vi "main_real-time control mouse 23.3.1.vi"() -> ()   [LabVIEW 2020]
uses:
  <vilib>/Analysis/3filter.llb/Filter Passband Type.ctl
  <vilib>/Analysis/NI_AALBase.lvlib
  <vilib>/Analysis/3filter.llb/Butterworth Filter (DBL).vi
  <vilib>/express/express analysis/Spectral/XNode/ExpressSpectralMeasurementsBlockNode.xnode
  <vilib>/express/express analysis/Spectral/Block/exnSpectralBlock spectral measurements power poly.vi
  <vilib>/Analysis/NI_AALPro.lvlib
  <vilib>/Analysis/NI_AAL_SigProc.lvlib
  <vilib>/Utility/file.llb/Write Delimited Spreadsheet (DBL).vi
  <vilib>/express/express analysis/Spectral/Block/exnSpectralBlock spectral measurements power DDT.vi
panel:
  out "手势":string
  in  "训练——手势":string
  out "卡尔曼滤波":cluster{"Y":dbl[], "Y":dbl[]}[](graph)
  out "通道1":dynamicdata(graph)
  out "XY Graph 2":cluster{"Y":dbl[], "Y":dbl[]}[](graph) caption="ML_集成树"
  in  "训练——位置":dbl
  out "数值":dbl
  out "采样点 2":dbl
  out "采样点":dbl
  out "ToF 2(cm)":dbl
  out "ToF 1(cm)":dbl
  out "有手势":bool
  out "最大值 1":dbl
  out "最大值2":dbl
  out "波形图 2":dbl[](graph)
  out "余数 2":dbl
  out "循环 2":dbl
  out "波形图":dbl[](graph)
  out "通道1_去环境噪声":dbl[](graph)
  out "通道2_去环境+滤波":dbl[](graph)
  out "频谱2":dynamicdata(graph)
  out "通道1_滤波":dbl[](graph)
  out "通道2_滤波":dbl[](graph)
  out "激励信号":dynamicdata(graph)
  out "通道2":dynamicdata(graph)
  in  "停止":bool
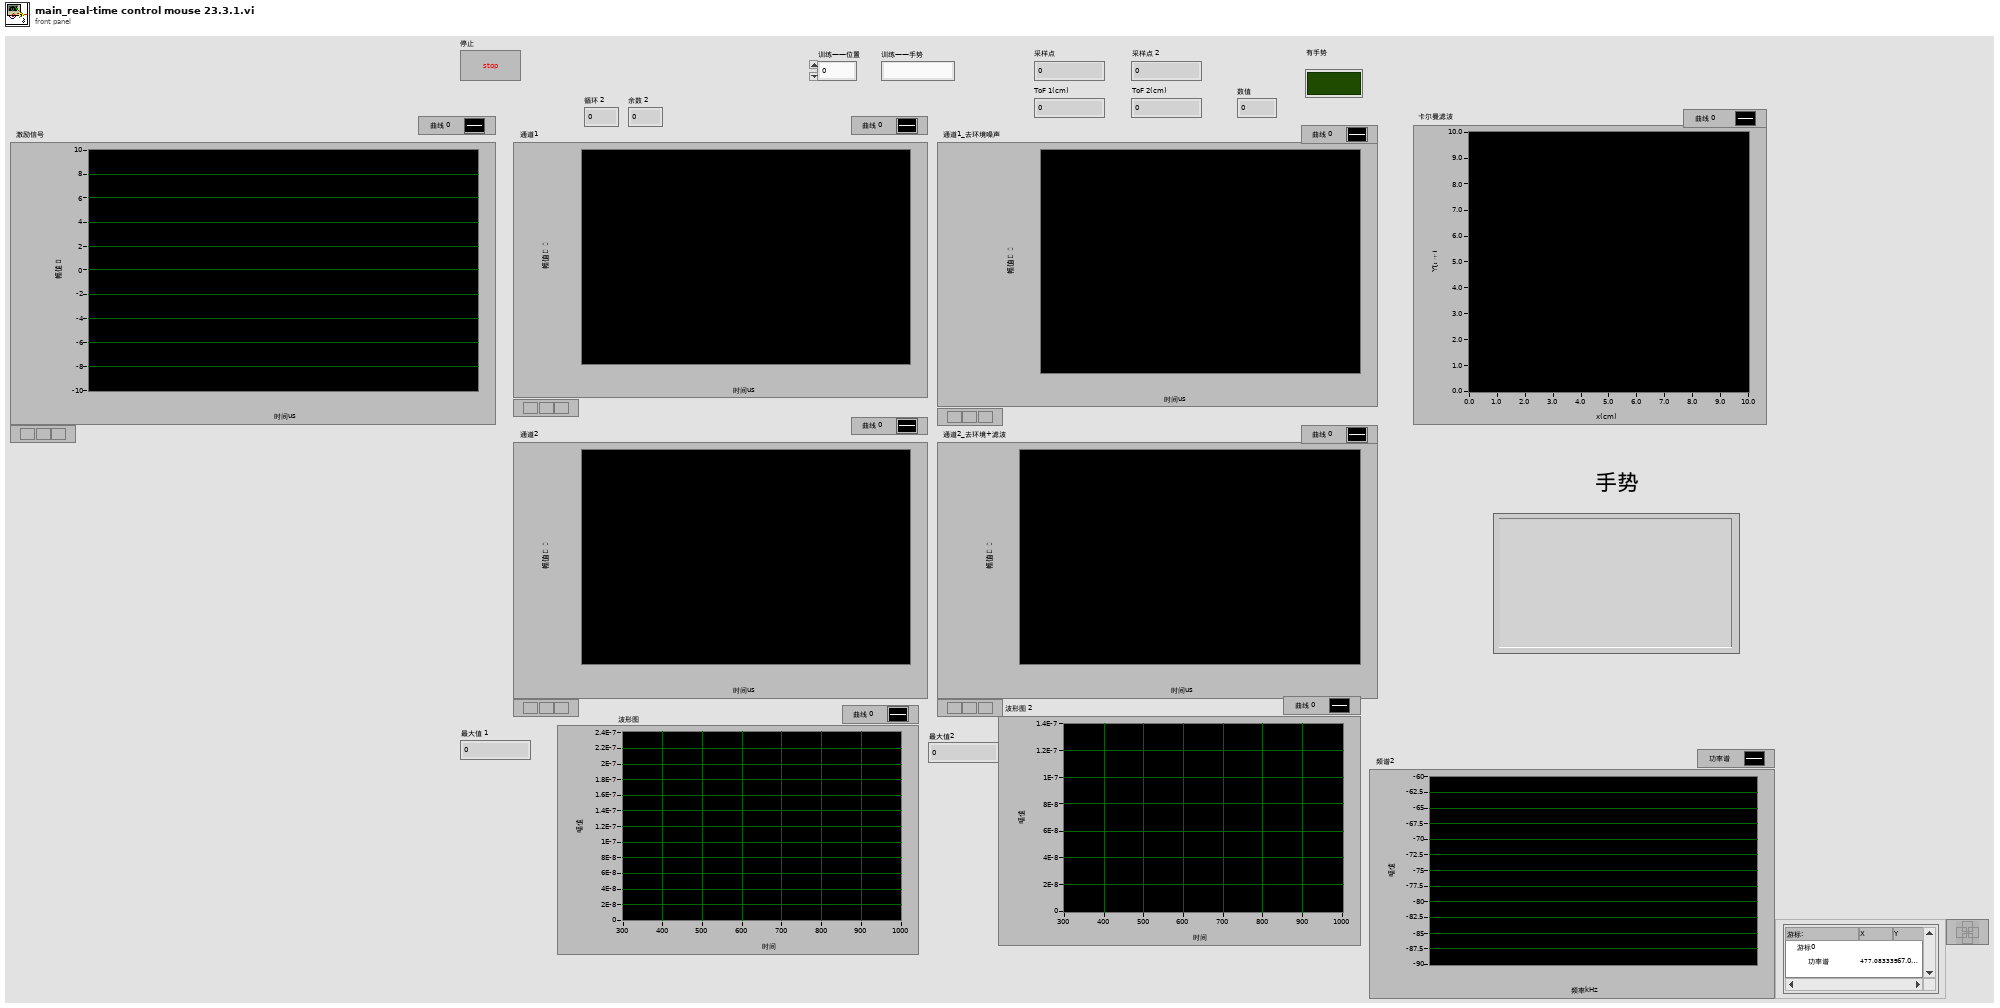
[diagram p1: front panel]
types:
  T1 = typedef "NI_AALBase.lvlib/Filter Passband Type.ctl" = enum32{"Lowpass", "Highpass", "Bandpass", "Bandstop"}
  T2 = cluster{"averaging mode":u16, "weighting mode":u16, "number of averages":u32}
  T3 = cluster{"dB On (F)":bool, "unwrap phase (F)":bool, "convert to degree (F)":bool}
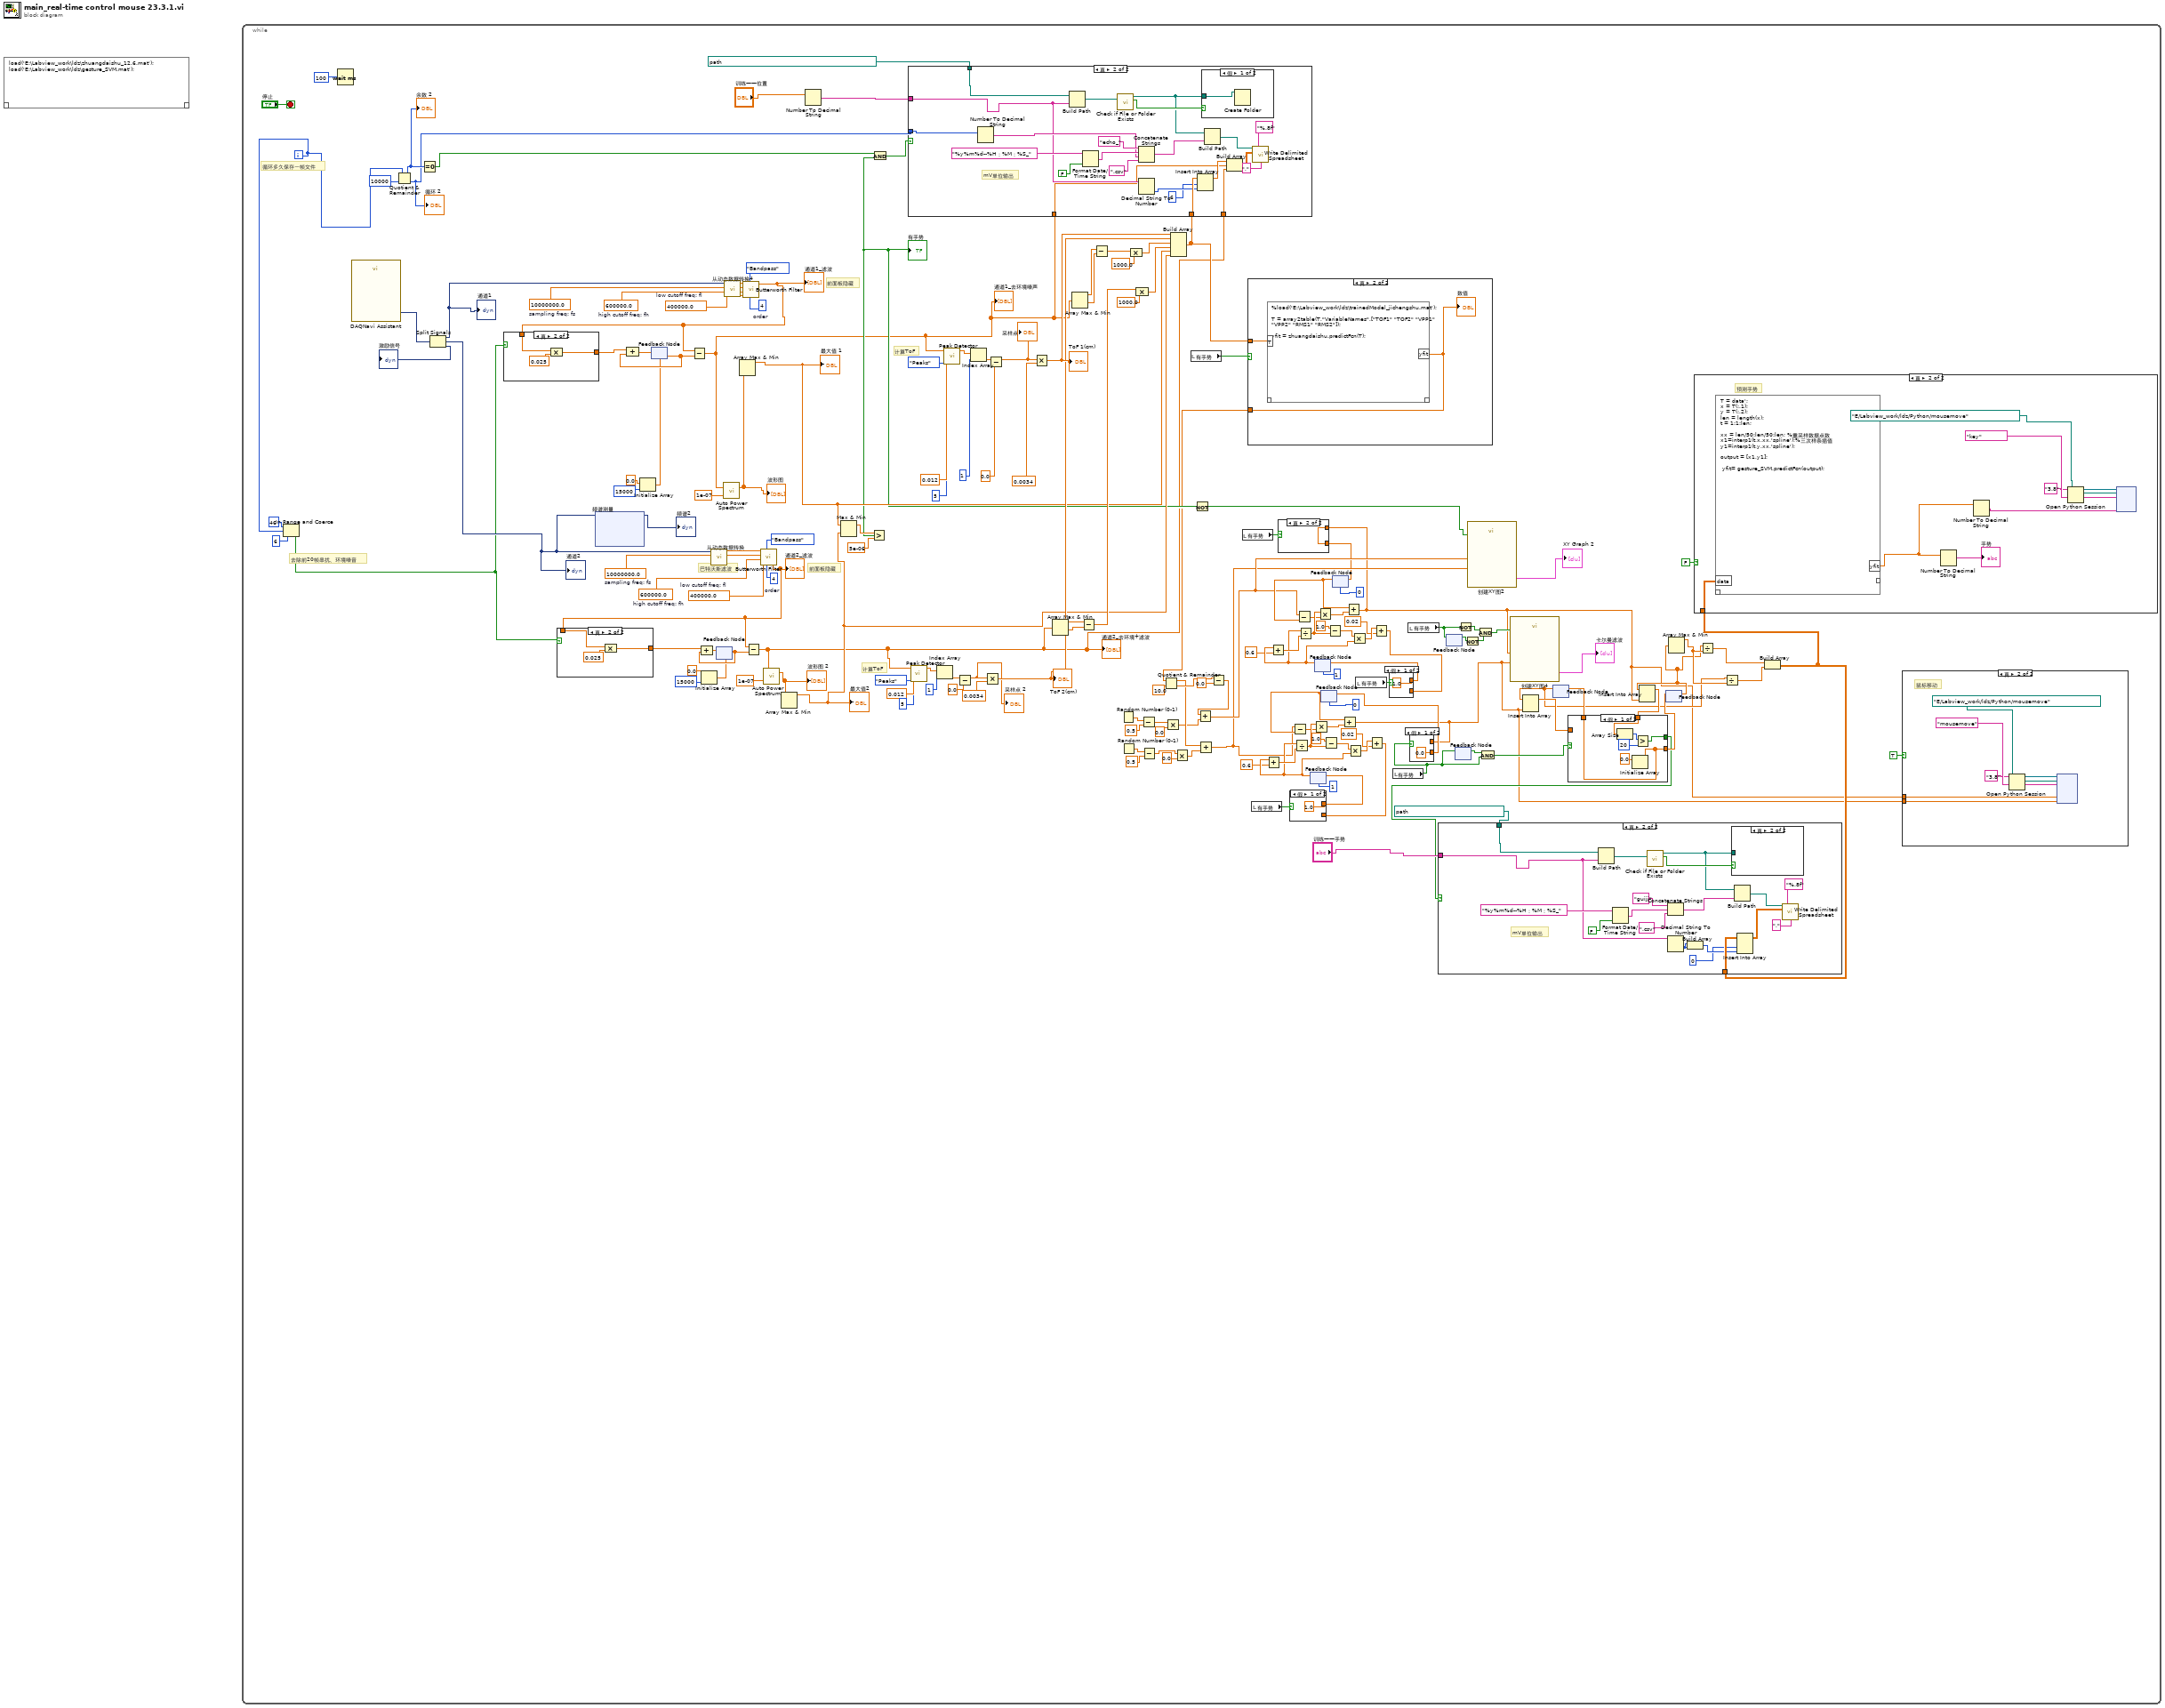
[diagram p0: block diagram]
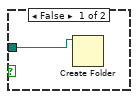
[diagram p5: hidden frame]
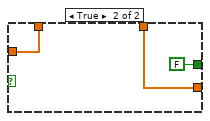
[diagram p6: hidden frame]
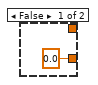
[diagram p10: hidden frame]
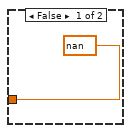
[diagram p11: hidden frame]
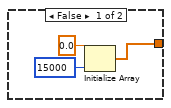
[diagram p14: hidden frame]
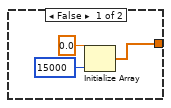
[diagram p15: hidden frame]
diagram:
  n1 = script code="load('E:\\Labview_work\\ldz\\zhuangdaishu_12.6.mat');\nload('E:\\Labview_work\\ldz\\gesture_SVM.mat');"() -> ()  [unwired: 1 in, 1 out]
  n2 = while {
    i -> [w134]
    stop <- "停止" stop-if-true
    w156 = 400000.0  # low cutoff freq: fl
    w160 = 600000.0  # high cutoff freq: fh
    w159 = 10000000.0  # sampling freq: fs
    w161 = 4  # order
    w167 = 400000.0  # low cutoff freq: fl
    w166 = 600000.0  # high cutoff freq: fh
    w165 = 10000000.0  # sampling freq: fs
    w168 = 4  # order
    # "计算ToF"
    # "计算ToF"
    # "前面板隐藏"
    # "前面板隐藏"
    # "去除前20帧串扰、环境噪音"
    # "循环多久保存一帧文件"
    # "巴特沃斯滤波"
    n3 = In Range and Coerce(upper limit=46 ("上限"), x=w134, lower limit=6 ("下限")) -> (In Range?=w138:bool)  [unwired: 1 out]
    n4 = Wait (ms)(milliseconds to wait=100) -> ()  [unwired: 1 out]
    n5 = call "DAQNavi Assistant"() -> ("data out(DDT)"=w154:dynamicdata)  [unwired: 6 in, 21 out]
    n6 = Quotient & Remainder(x=w134, y=10000) -> (x-y*floor(x/y)=w136:i32, floor(x/y)=w135:i32)
    "循环 2" <- w135
    "余数 2" <- w136
    n7 = Equal To 0?(x=w136) -> (x = 0?=w125:bool)
    n8 = Split Signals(w154) -> (w90:dynamicdata, w155:dynamicdata, →"激励信号":dynamicdata)  [unwired: 3 in]
    "通道2" <- w155
    "通道1" <- w90
    n9 = xnode "频谱测量"("信号"=w155) -> ("功率谱"=→"频谱2":dynamicdata)  [unwired: 1 in, 1 out]
    n10 = Initialize Array(0.0 ("元素"), 15000 ("维数大小")) -> (w142:dbl[])
    n11 = feedback #1(w142) -> (w144:dbl[])
    n12 = Initialize Array(0.0 ("元素"), 15000 ("维数大小")) -> (w150:dbl[])
    n13 = call "从动态数据转换"("Dynamic Data Type"=w155) -> ("Array"=w163:dbl[])  [unwired: 3 in]
    n14 = feedback #2(w150) -> (w151:dbl[])
    n15 = call "从动态数据转换4"("Dynamic Data Type"=w90) -> ("Array"=w157:dbl[])  [unwired: 3 in]
    n16 = call-poly <vilib>:"Butterworth Filter.vi"("order"=w161, "filter type"=Filter_Passband_Type."Bandpass", "low cutoff freq: fl"=w156, "high cutoff freq: fh"=w160, "sampling freq: fs"=w159, "X"=w157) -> ("Filtered X"=w89:dbl[])  [unwired: 2 in, 1 out]
    "通道1_滤波" <- w89
    n17 = case shown="真" w138 {
      tunnel: w89 -> [_ w251]
      tunnel: [w248 w253] -> w146
      frame False {
        n18 = Initialize Array(0.0 ("元素"), 15000 ("维数大小")) -> (w248:dbl[])
      }
      frame True {
        n19 = Compound Arithmetic op=MULTIPLY(w251, 0.025) -> (w253:dbl[])
      }
    }
    n20 = Compound Arithmetic op=ADD(w146, w144) -> (w145:dbl[])
    n21 = feedback-in #1(w145) -> ()
    n22 = Subtract(x=w89, y=w144) -> (x-y=w2:dbl[])
    "通道1_去环境噪声" <- w2
    n23 = call <vilib>:"Auto Power Spectrum.vi"("dt"=1e-07, "Signal (V)"=w2) -> ("Power Spectrum (V^2 rms)"=w128:dbl[])  [unwired: 1 out]
    "波形图" <- w128
    n24 = Array Max & Min(array=w128) -> (max value=w97:dbl)  [unwired: 3 out]
    "最大值 1" <- w97
    n25 = call-poly <vilib>:"Butterworth Filter.vi"("order"=w168, "filter type"=Filter_Passband_Type."Bandpass", "low cutoff freq: fl"=w167, "high cutoff freq: fh"=w166, "sampling freq: fs"=w165, "X"=w163) -> ("Filtered X"=w147:dbl[])  [unwired: 2 in, 1 out]
    "通道2_滤波" <- w147
    n26 = case shown="真" w138 {
      tunnel: w147 -> [_ w259]
      tunnel: [w254 w258] -> w153
      frame False {
        n27 = Initialize Array(0.0 ("元素"), 15000 ("维数大小")) -> (w254:dbl[])
      }
      frame True {
        n28 = Compound Arithmetic op=MULTIPLY(w259, 0.025) -> (w258:dbl[])
      }
    }
    n29 = Compound Arithmetic op=ADD(w153, w151) -> (w152:dbl[])
    n30 = feedback-in #2(w152) -> ()
    n31 = Subtract(x=w147, y=w151) -> (x-y=w1:dbl[])
    "通道2_去环境+滤波" <- w1
    n32 = call <vilib>:"Auto Power Spectrum.vi"("dt"=1e-07, "Signal (V)"=w1) -> ("Power Spectrum (V^2 rms)"=w129:dbl[])  [unwired: 1 out]
    "波形图 2" <- w129
    n33 = Array Max & Min(array=w129) -> (max value=w96:dbl)  [unwired: 3 out]
    "最大值2" <- w96
    n34 = Number To Decimal String(number="训练——位置") -> (decimal integer string=w92:string)  [unwired: 1 in]
    n35 = Max & Min(x=w97, y=w96) -> (max(x,y)=w127:dbl)  [unwired: 1 out]
    n36 = Greater?(x=w127, y=5e-06) -> (0:w95:bool)
    "有手势" <- w95
    n37 = And(x=w125, y=w95) -> (x .and. y?=w124:bool)
    n38 = call <vilib>:"Peak Detector.vi"("peaks/valleys"=enum32{"Peaks", "Valleys"}."Peaks", "width"=5, "threshold"=0.012, "X"=w1) -> ("Locations"=w115:dbl[])  [unwired: 3 in, 4 out]
    n39 = Index Array(array=w115, index=1 ("索引")) -> (element=w85:dbl)
    n40 = call <vilib>:"Peak Detector.vi"("peaks/valleys"=enum32{"Peaks", "Valleys"}."Peaks", "width"=5, "threshold"=0.012, "X"=w2) -> ("Locations"=w120:dbl[])  [unwired: 3 in, 4 out]
    n41 = Subtract(x=w85, y=0.0) -> (x-y=w86:dbl)
    "采样点 2" <- w86
    n42 = Index Array(array=w120, index=1 ("索引")) -> (element=w113:dbl)
    n43 = Multiply(x=w86, y=0.0034) -> (x*y=w108:dbl)
    "ToF 2(cm)" <- w108
    n44 = Subtract(x=w113, y=0.0) -> (x-y=w88:dbl)
    "采样点" <- w88
    n45 = Multiply(x=w88, y=0.0034) -> (x*y=w109:dbl)
    "ToF 1(cm)" <- w109
    n46 = Array Max & Min(array=w1) -> (max value=w100:dbl, min value=w99:dbl)  [unwired: 2 out]
    n47 = Array Max & Min(array=w2) -> (max value=w104:dbl, min value=w103:dbl)  [unwired: 2 out]
    n48 = Subtract(x=w100, y=w99) -> (x-y=w101:dbl)
    n49 = Subtract(x=w104, y=w103) -> (x-y=w102:dbl)
    n50 = Random Number (0-1)() -> (number: 0 to 1=w80:dbl)
    n51 = Random Number (0-1)() -> (number: 0 to 1=w77:dbl)
    n52 = Compound Arithmetic op=MULTIPLY(w102, 1000.0) -> (w106:dbl)
    n53 = Compound Arithmetic op=MULTIPLY(w101, 1000.0) -> (w98:dbl)
    n54 = Subtract(x=w80, y=0.5) -> (x-y=w74:dbl)
    n55 = Subtract(x=w77, y=0.5) -> (x-y=w69:dbl)
    n56 = Multiply(x=w74, y=0.0) -> (x*y=w73:dbl)
    n57 = Build Array(w109, w108, w106, w98, w97, w96) -> (w94:dbl[])
    n58 = case shown="真" w124 {
      tunnel: w135 -> [_ w237]
      tunnel: path "E:/Labview_work/ldz/数据/3.7/波形数据" ("路径") -> [_ w234]
      tunnel: w94 -> [_ w232]
      tunnel: w92 -> [_ w228]
      tunnel: w2 -> [_ w226]
      tunnel: w1 -> [_ w225]
      frame False {
      }
      frame True {
        # "mV单位输出"
        n59 = Number To Decimal String(number=w237) -> (decimal integer string=w236:string)  [unwired: 1 in]
        n60 = Build Path(base path=w234, name or relative path=w228) -> (appended path=w241:path)
        n61 = Format Date/Time String ("格式化日期/时间字符串")(time format string (%c)="%y%m%d--%H：%M：%S_", UTC format=FALSE) -> (date/time string=w243:string)  [unwired: 1 in]
        n62 = call <vilib>:"Check if File or Folder Exists.vi"("path"=w241) -> ("file or folder exists?"=w240:bool, "dup path"=w229:path)  [unwired: 8 in, 1 out]
        n63 = Concatenate Strings("echo_" ("字符串"), w243, w236, ".csv" ("字符串")) -> (w245:string)
        n64 = Decimal String To Number(string=w228) -> (number=w231:i32)  [unwired: 2 in, 1 out]
        n65 = Insert Into Array(array=w232, index=6 ("索引"), new element=w231) -> (w227:dbl[])
        n66 = case shown="假" w240 {
          tunnel: w229 -> [w247 _]
          frame False {
            n67 = Create Folder(path (use dialog)=w247) -> ()  [unwired: 2 in, 3 out]
          }
          frame True {
          }
        }
        n68 = Build Path(base path=w229, name or relative path=w245) -> (appended path=w244:path)
        n69 = Build Array(w227, w226, w225) -> (w224:dbl[][])
        n70 = call-poly <vilib>:"Write Delimited Spreadsheet.vi"("file path (dialog if empty)"=w244, "format (%.3f)"="%.8f", "2D data"=w224, "delimiter (\\t)"="," ("delimiter (\\t)")) -> ()  [unwired: 10 in, 2 out]
      }
    }
    n71 = Multiply(x=w69, y=0.0) -> (x*y=w70:dbl)
    n72 = local read "有手势"() -> (w39:bool)
    n73 = Not(x=w95) -> (.not. x?=w24:bool)
    n74 = local read "有手势"() -> (w34:bool)
    n75 = case shown="真" w39 {
      tunnel: w94 -> [_ w223]
      tunnel: [nan w222] -> w42
      frame False {
      }
      frame True {
        n76 = script code="%load('E:\\Labview_work\\ldz\\trainedModel_jichengshu.mat');\n\nT = array2table(T,\"VariableNames\",[\"TOF1\" \"TOF2\" \"VPP1\" \"VPP2\" \"RMS1\" \"RMS2\"]);\n\nyfit = zhuangdaishu.predictFcn(T);" ("脚本节点")("T"=w223) -> ("yfit"=w222:dbl)  [unwired: 1 in, 1 out]
        "数值" <- w222
      }
    }
    n77 = Quotient & Remainder(x=w42, y=10.0) -> (x-y*floor(x/y)=w75:dbl, floor(x/y)=w82:dbl)
    n78 = Add(x=w75, y=w70) -> (x+y=w40:dbl)
    n79 = Subtract(x=w82, y=0.0) -> (x-y=w78:dbl)
    n80 = Add(x=w78, y=w73) -> (x+y=w41:dbl)
    n81 = local read "有手势"() -> (w32:bool)
    n82 = feedback #3(1) -> (w48:dbl)
    n83 = Add(x=w48, y=0.6) -> (x+y=w55:dbl)
    n84 = Divide(x=w48, y=w55) -> (x/y=w53:dbl)
    n85 = feedback #4(1) -> (w61:dbl)
    n86 = Add(x=w61, y=0.6) -> (x+y=w68:dbl)
    n87 = Divide(x=w61, y=w68) -> (x/y=w66:dbl)
    n88 = feedback #5(0) -> (w47:dbl)
    n89 = Subtract(x=w40, y=w47) -> (x-y=w52:dbl)
    n90 = Multiply(x=w53, y=w52) -> (x*y=w51:dbl)
    n91 = Subtract(x=1.0, y=w53) -> (x-y=w50:dbl)
    n92 = Subtract(x=1.0, y=w66) -> (x-y=w63:dbl)
    n93 = feedback #6(0) -> (w60:dbl)
    n94 = Subtract(x=w41, y=w60) -> (x-y=w65:dbl)
    n95 = Multiply(x=w66, y=w65) -> (x*y=w64:dbl)
    n96 = Add(x=w47, y=w51) -> (x+y=w6:dbl)
    n97 = Add(x=w60, y=w64) -> (x+y=w7:dbl)
    n98 = case shown="真" w34 {
      tunnel: w7 -> [_ w220]
      tunnel: [0.0 w220] -> w33
      frame False {
      }
      frame True {
      }
    }
    n99 = feedback-in #6(w33) -> ()
    n100 = Multiply(x=w50, y=w48) -> (x*y=w49:dbl)
    n101 = Multiply(x=w63, y=w61) -> (x*y=w62:dbl)
    n102 = local read "有手势"() -> (w27:bool)
    n103 = Add(x=w49, y=0.02) -> (x+y=w31:dbl)
    n104 = case shown="假" w32 {
      tunnel: w31 -> [_ w218]
      tunnel: [1.0 w218] -> w30
      frame False {
      }
      frame True {
      }
    }
    n105 = feedback-in #3(w30) -> ()
    n106 = Add(x=w62, y=0.02) -> (x+y=w29:dbl)
    n107 = case shown="假" w27 {
      tunnel: w29 -> [_ w216]
      tunnel: [1.0 w216] -> w28
      frame False {
      }
      frame True {
      }
    }
    n108 = feedback-in #4(w28) -> ()
    n109 = local read "有手势"() -> (w5:bool)
    n110 = local read "有手势"() -> (w25:bool)
    n111 = case shown="假" w5 {
      tunnel: w6 -> [_ w214]
      tunnel: [0.0 w214] -> w26
      frame False {
      }
      frame True {
      }
    }
    n112 = feedback-in #5(w26) -> ()
    n113 = feedback-in #7(w25) -> ()
    n114 = feedback #7() -> (w36:bool)  [unwired: 1 in]
    n115 = feedback #8() -> (w9:bool)  [unwired: 1 in]
    n116 = feedback-in #8(w5) -> ()
    n117 = Not(x=w25) -> (.not. x?=w38:bool)
    n118 = Not(x=w36) -> (.not. x?=w35:bool)
    n119 = call "创建XY图2"("Reset"=w24, "Y Input"=w40, "X Input"=w41) -> ("XY Graph"=→"XY Graph 2":cluster{"X":dbl[], "Y":dbl[]}[])  [unwired: 7 in, 1 out]
    n120 = And(x=w38, y=w35) -> (x .and. y?=w37:bool)
    n121 = And(x=w9, y=w5) -> (x .and. y?=w8:bool)
    n122 = call "创建XY图4"("Reset"=w37, "Y Input"=w6, "X Input"=w7) -> ("XY Graph"=→"卡尔曼滤波":cluster{"X":dbl[], "Y":dbl[]}[])  [unwired: 7 in, 1 out]
    n123 = feedback #9() -> (w14:dbl[])  [unwired: 1 in]
    n124 = Insert Into Array(array=w14, new element=w6) -> (w19:dbl[])  [unwired: 1 in]
    n125 = feedback #10() -> (w15:dbl[])  [unwired: 1 in]
    n126 = Insert Into Array(array=w15, new element=w7) -> (w20:dbl[])  [unwired: 1 in]
    n127 = case shown="假" w8 {
      tunnel: w20 -> [w208 w212]
      tunnel: [w204 w212] -> w16
      tunnel: [w205 FALSE] -> w10
      tunnel: w19 -> [_ w210]
      tunnel: [w204 w210] -> w17
      frame False {
        n128 = Array Size(array=w208) -> (size(s)=w207:i32)
        n129 = Initialize Array(0.0 ("元素")) -> (w204:dbl[])  [unwired: 1 in]
        n130 = Greater?(x=w207, y=20) -> (0:w205:bool)
      }
      frame True {
      }
    }
    n131 = feedback-in #9(w17) -> ()
    n132 = feedback-in #10(w16) -> ()
    n133 = Array Max & Min(array=w15) -> (max value=w18:dbl)  [unwired: 3 out]
    n134 = Divide(x=w15, y=w18) -> (x/y=w13:dbl[])
    n135 = Divide(x=w14, y=w18) -> (x/y=w12:dbl[])
    n136 = Build Array(w13, w12) -> (w11:dbl[][])
    n137 = case shown="真" w10 {
      tunnel: path "E:/Labview_work/ldz/数据/3.7/手势" ("路径") -> [_ w193]
      tunnel: "训练——手势" -> [_ w190]
      tunnel: w11 -> [_ w188]
      frame False {
      }
      frame True {
        # "mV单位输出"
        n138 = Build Path(base path=w193, name or relative path=w190) -> (appended path=w197:path)
        n139 = Format Date/Time String ("格式化日期/时间字符串")(time format string (%c)="%y%m%d--%H：%M：%S_", UTC format=FALSE) -> (date/time string=w199:string)  [unwired: 1 in]
        n140 = call <vilib>:"Check if File or Folder Exists.vi"("path"=w197) -> ("file or folder exists?"=w196:bool, "dup path"=w191:path)  [unwired: 8 in, 1 out]
        n141 = Concatenate Strings("guiji" ("字符串"), w199, ".csv" ("字符串")) -> (w201:string)
        n142 = Decimal String To Number(string=w190) -> (number=w187:i32)  [unwired: 2 in, 1 out]
        n143 = Build Array(w187, w187) -> (w186:i32[])
        n144 = case shown="真" w196 {
          tunnel: w191 -> [w203 _]
          frame False {
            n145 = Create Folder(path (use dialog)=w203) -> ()  [unwired: 2 in, 3 out]
          }
          frame True {
          }
        }
        n146 = Build Path(base path=w191, name or relative path=w201) -> (appended path=w200:path)
        n147 = Insert Into Array(array=w188, index (col)=0 ("索引"), new element=w186) -> (w184:dbl[][])  [unwired: 1 in]
        n148 = call-poly <vilib>:"Write Delimited Spreadsheet.vi"("file path (dialog if empty)"=w200, "format (%.3f)"="%.8f", "2D data"=w184, "delimiter (\\t)"="," ("delimiter (\\t)")) -> ()  [unwired: 10 in, 2 out]
      }
    }
    n149 = case shown="真" FALSE {
      tunnel: w11 -> [_ w183]
      frame False {
      }
      frame True {
        # "预测手势"
        n150 = script code="T = data';\nx = T(:,1);\ny = T(:,2);\nlen = length(x);\nt = 1:1:len;\n\nxx = len/50:len/50:len; %重采样数据点数\nx1=interp1(t,x,xx,'spline');%三次样条插值\ny1=interp1(t,y,xx,'spline');\n\noutput = [x1,y1];\n\n yfit= gesture_SVM.predictFcn(output);"("data"=w183) -> ("yfit"=w178:dbl)  [unwired: 1 in, 1 out]
        n151 = Number To Decimal String(number=w178) -> (decimal integer string=→"手势":string)  [unwired: 1 in]
        n152 = Number To Decimal String(number=w178) -> (decimal integer string=w177:string)  [unwired: 1 in]
        n153 = Open Python Session(python version="3.8" ("Python版本")) -> (session out=w179:refnum<k35>)  [unwired: 2 in, 1 out]
        n154 = node(w179, path "E:/Labview_work/ldz/Python/mousemove" ("路径"), "key" ("字符串"), w177) -> ()  [unwired: 4 in, 4 out]
      }
    }
    n155 = case shown="真" TRUE {
      tunnel: w7 -> [_ w171]
      tunnel: w6 -> [_ w170]
      frame False {
      }
      frame True {
        # "鼠标移动"
        n156 = Open Python Session(python version="3.8" ("Python版本")) -> (session out=w172:refnum<k35>)  [unwired: 2 in, 1 out]
        n157 = node(w172, path "E:/Labview_work/ldz/Python/mousemove" ("路径"), "mousemove" ("字符串"), w171, w170) -> ()  [unwired: 5 in, 4 out]
      }
    }
  }
